vi "FPExpContro.vi"(0 "Data In":T6 caption="Données en entrée", 2 "Display State In":T4 caption="État d'affichage en entrée", 3 "Container State":T5 caption="État du conteneur") -> (6 "Data Out":T6 caption="Données en sortie", 7 "Display State Out":T4 caption="État d'affichage en sortie", 8 "Action":T3)   [LabVIEW 2019, in "ControlExpControl.xctl"]
uses:
  ControlExpControl.xctl
  controls/xxx.ctl
  DataExpControl.ctl
  <vilib>/_xctls/Container State.ctl
  ExpControl.ctl
  <vilib>/_xctls/Action.ctl
  controls/SliderSDII.ctl
  <vilib>/_xctls/XControlSupport.lvlib
panel:
  in  "Aq contol":enum32{"fixed", "automatic", "fixed-auto"}(radio)
  in  "# par point":i32=10 min=1 max=50 step=1
  in  "times slider":T1={-0.46341463414634143, 0.46341463414634154} scale=-1.0..1.0 scale format="%#.1f"
  in  "Wavelength fix":dbl[unit]=6.4e-07 caption="wave fix"
  out "Delays":cluster{i32[], "array w/ subset deleted":dbl[]}(graph)
  in  "Load table":bool
  in  "Table path":path=path "C:/Users/Sergey Denisov/Dropbox/LCP/Soft/LabVIEW/TRANCON-2016/delay/main-delay.txt"
  in  "OZ, ps":dbl[unit]=-2.5e-10 min=-5e-09 max=9e-09
  in  "#":i32=100 min=1 step=1
  in  "Step, ps":T2=15.0 min=-100.0 max=1000.0 step=1.0
  in  "Real zero, ps":dbl[unit]=4.75e-10
  in  "remake":bool
  out "status":u8(slide) scale=0.0..100.0
  # "1. Déposez ici les commandes qui constituent l'apparence de la commandeX.\n\n2. Redimensionnez la fenêtre pour l'ajuster aux commandes.\n\n3. Si la taille de la commandeX est fixe, utilisez la page Propriétés du VI ->Apparence de la fenêtre pour empêcher la fenêtre de se redimensionner.\n\n4. Si vous voulez que les commandes se redimensionnent automatiquement quand la commandeX se redimensionne, sélectionnez l'option \"Mettre à l'échelle tous les objets de la face-avant lors du redimensionnement de la fenêtre\" sur la page Fichier ->Propriétés du VI ->Taille de la fenêtre.\n\n5. Affichez le diagramme et traitez les événements des commandes de cette face-avant."
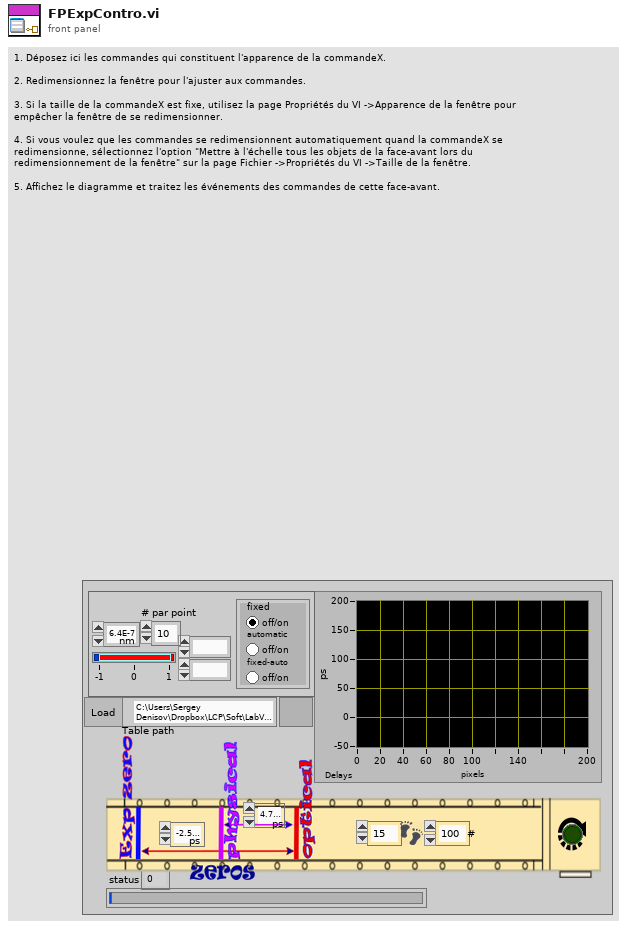
[diagram p1: front panel]
types:
  T1 = typedef "SliderSDII.ctl" = cluster{dbl, dbl}
  T2 = typedef "xxx.ctl" = dbl
  T3 = typedef "XControlSupport.lvlib/Action.ctl" = cluster{"Data Changed?":bool, "State Changed?":bool, "Action Name":string}
  T4 = typedef "ControlExpControl.xctl/ExpControl.ctl" = cluster{"Delays":dbl[], "zero delay":dbl, "optical  zero":dbl, "#point":dbl, "step":dbl, "#parpoint":dbl, "Aq contol":enum32{"fixed", "automatic", "fixed-auto"}, "fix wavelength":dbl, "remake":bool, "Table path":path, "Delays 2":cluster{i32[], "array w/ subset deleted":dbl[]}}
  T5 = typedef "XControlSupport.lvlib/Container State.ctl" = cluster{"Indicator?":bool, "Run Mode?":bool, " Refnum":refnum<vi>}
  T6 = typedef "ControlExpControl.xctl/DataExpControl.ctl" = dbl[]
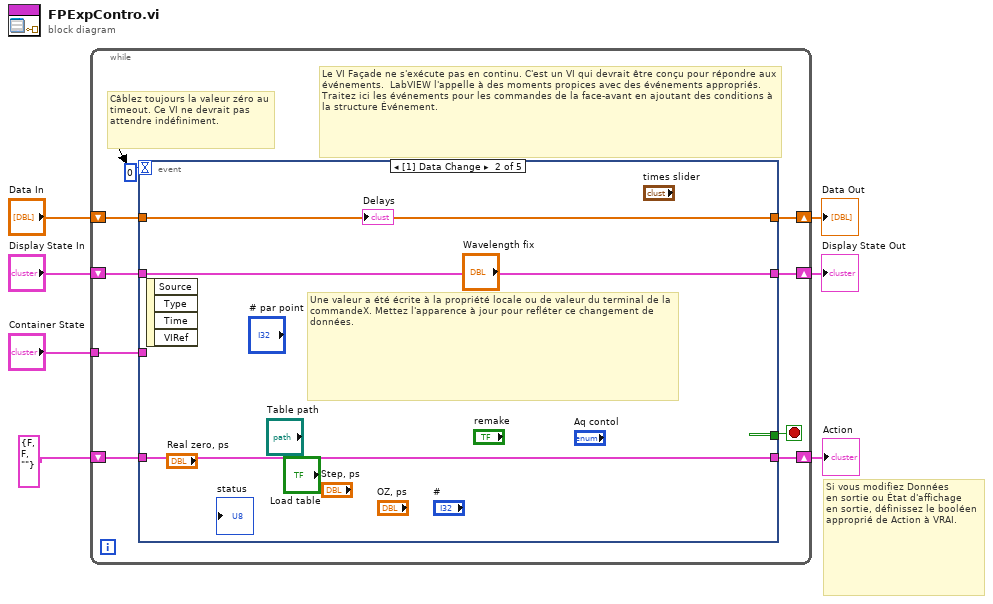
[diagram p0: block diagram]
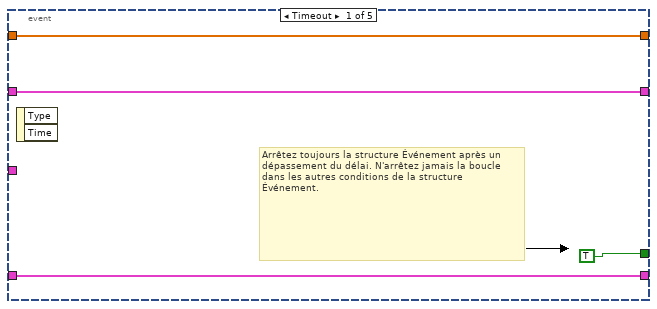
[diagram p2: hidden frame]
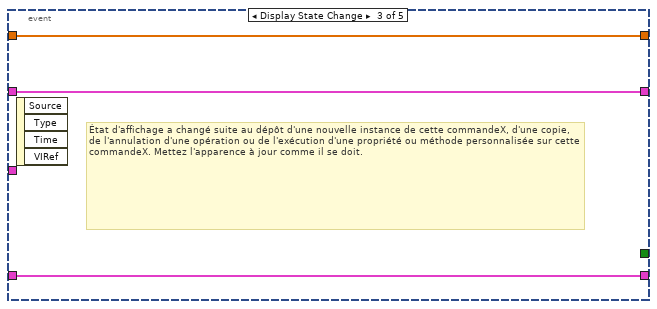
[diagram p3: hidden frame]
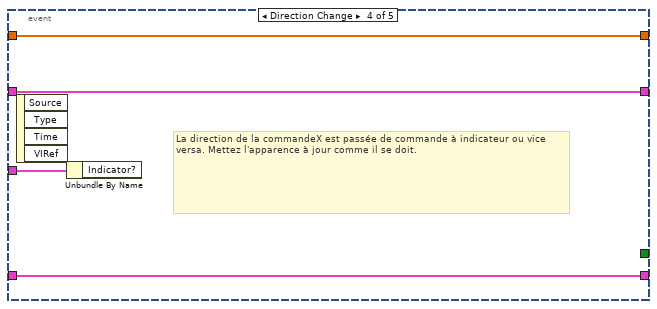
[diagram p4: hidden frame]
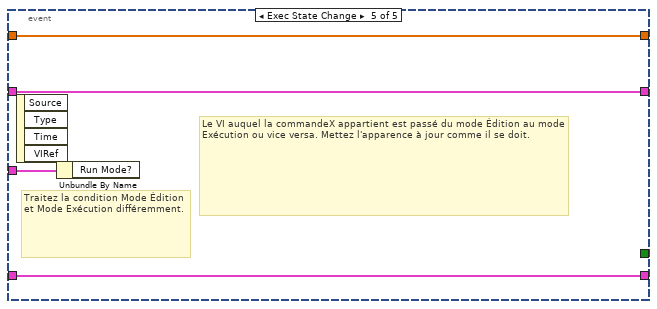
[diagram p5: hidden frame]
diagram:
  # "Si vous modifiez Données\nen sortie ou État d'affichage\nen sortie, définissez le booléen\napproprié de Action à VRAI."
  n1 = while {
    shift-right: [w15] -> w4
    shift-left: "Display State In" -> [w16]
    tunnel: "Container State" -> [w12]
    shift-right: [w10] -> w7
    shift-left: "Data In" -> [w11]
    shift-right: [w8] -> w2
    shift-left: T3 {"Data Changed?"=FALSE, "State Changed?"=FALSE, "Action Name"=""} ("Action") -> [w9]
    stop <- w14 stop-if-true
    # "Le VI Façade ne s'exécute pas en continu. C'est un VI qui devrait être conçu pour répondre aux événements.  LabVIEW l'appelle à des moments propices avec des événements appropriés. Traitez ici les événements pour les commandes de la face-avant en ajoutant des conditions à la structure Événement."
    # "Câblez toujours la valeur zéro au timeout. Ce VI ne devrait pas attendre indéfiniment."
    n2 = event shown="[1] Data Change" {
      selector: _ -> [_ _ _ _ _]
      dyn-events: _ -> [_ _ _ _ _]
      timeout: 0 -> [_ _ _ _ _]
      tunnel: w16 -> [w18 w22 w26 w29 w33]
      tunnel: [w18 w22 w26 w29 w33] -> w15
      tunnel: [TRUE _ _ _ _] -> w14
      tunnel: w12 -> [_ _ _ w30 w34]
      tunnel: w11 -> [w17 w23 w25 w28 w32]
      tunnel: [w17 w23 w25 w28 w32] -> w10
      tunnel: [w19 w21 w24 w27 w31] -> w8
      tunnel: w9 -> [w19 w21 w24 w27 w31]
      event Timeout {
        # "Arrêtez toujours la structure Événement après un dépassement du délai. N'arrêtez jamais la boucle dans les autres conditions de la structure Événement."
        n3 = event-data() -> ()  [unwired: 1 in, 2 out]
      }
      event Data Change {
        # "Une valeur a été écrite à la propriété locale ou de valeur du terminal de la commandeX. Mettez l'apparence à jour pour refléter ce changement de données."
        n4 = event-data() -> ()  [unwired: 1 in, 4 out]
      }
      event Display State Change {
        # "État d'affichage a changé suite au dépôt d'une nouvelle instance de cette commandeX, d'une copie, de l'annulation d'une opération ou de l'exécution d'une propriété ou méthode personnalisée sur cette commandeX. Mettez l'apparence à jour comme il se doit."
        n5 = event-data() -> ()  [unwired: 1 in, 4 out]
      }
      event Direction Change {
        # "La direction de la commandeX est passée de commande à indicateur ou vice versa. Mettez l'apparence à jour comme il se doit."
        n6 = event-data() -> ()  [unwired: 1 in, 4 out]
        n7 = Unbundle By Name(w30) -> ()  [unwired: 1 out]
      }
      event Exec State Change {
        # "Le VI auquel la commandeX appartient est passé du mode Édition au mode Exécution ou vice versa. Mettez l'apparence à jour comme il se doit."
        # "Traitez la condition Mode Édition et Mode Exécution différemment."
        n8 = event-data() -> ()  [unwired: 1 in, 4 out]
        n9 = Unbundle By Name(w34) -> ()  [unwired: 1 out]
      }
    }
  }
  "Display State Out" <- w4
  "Data Out" <- w7
  "Action" <- w2
